vi "RampAcceleration.vi"(7 "Low Pass Filter Average Length\n(.003-.007 Rec)":dbl=0.05, 10 "Joystick Input":dbl(slide) scale=-1.0..1.0) -> (3 "Motor Output":dbl)   [LabVIEW 2013]
uses:
  <vilib>/ptbypt/NI_PtbyPt.lvlib
  <vilib>/addons/control/pid/NI_PID_pid.lvlib
  <vilib>/addons/control/pid/pid.llb/PID Output Rate Limiter (DBL).vi
panel:
  in  "output rate (EGU/min)":dbl=200.0
  in  "Average Filter Sample Length":i32=10
  out "Input to Motor":T1(graph)={"Joystick Input"=0.0, "upper limit"=-1.761109083191672e-27, "upper limit"=0.0, "output"=0.0}
  # "Credit to Team 3005"
  # "Lower means less responsive curve\nHigher means quick, more responsive"
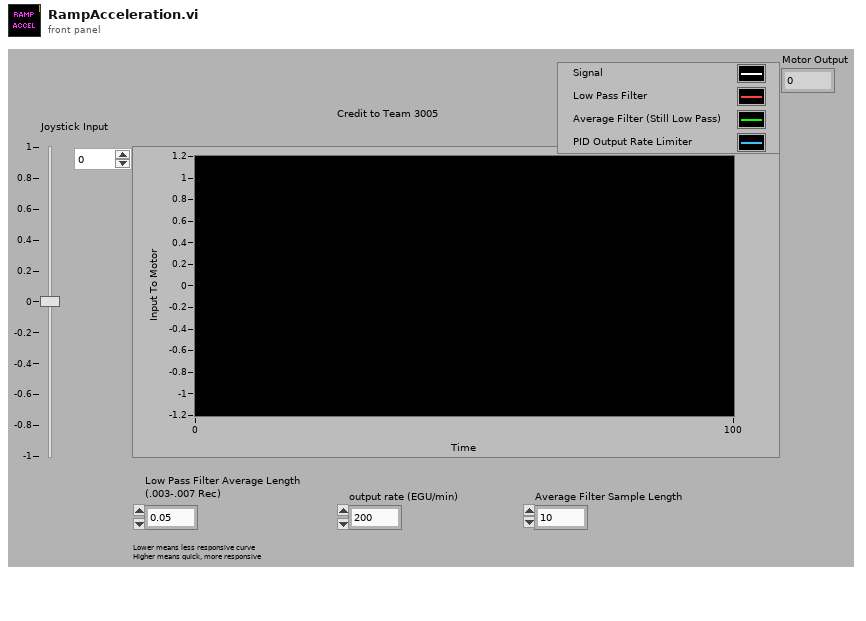
[diagram p1: front panel]
types:
  T1 = cluster{"Joystick Input":dbl, "upper limit":dbl, "upper limit":dbl, "output":dbl}
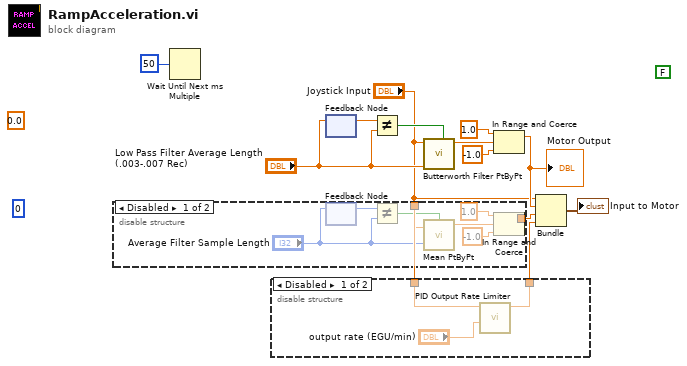
[diagram p0: block diagram]
diagram:
  (unwired) FALSE
  (unwired) 0 ("Average Filter Sample Length")
  (unwired) 0.0 ("Low Pass Filter Average Length")
  n1 = disable-structure shown="Disabled" {
    disable-tunnel: [w17 _] -> w6
    disable-tunnel: "Joystick Input" -> [w13 _]
    frame Disabled {
      n2 = feedback #1() -> (w16:i32)  [unwired: 1 in]
      n3 = feedback-in #1("Average Filter Sample Length") -> ()
      n4 = Not Equal?(x=w16, y="Average Filter Sample Length") -> (x != y?=w14:bool)
      n5 = call <vilib>:"Mean PtByPt.vi"("x"=w13, "sample length"="Average Filter Sample Length", "initialize"=w14) -> ("mean"=w18:dbl)  [unwired: 1 in, 1 out]
      n6 = In Range and Coerce(upper limit=1.0, x=w18, lower limit=-1.0) -> (coerced(x)=w17:dbl)  [unwired: 1 out]
    }
    frame Enabled {
    }
  }
  n7 = Wait Until Next ms Multiple(millisecond multiple=u32 50) -> ()  [unwired: 1 out]
  n8 = disable-structure shown="Disabled" {
    disable-tunnel: "Joystick Input" -> [w23 _]
    disable-tunnel: [w21 _] -> w1
    frame Disabled {
      n9 = call-poly <vilib>:"PID Output Rate Limiter.vi"("output rate (EGU/min)"="output rate (EGU/min)", "input (controller output)"=w23) -> ("output"=w21:dbl)  [unwired: 6 in, 1 out]
    }
    frame Enabled {
    }
  }
  n10 = feedback #2() -> (w5:dbl)  [unwired: 1 in]
  n11 = feedback-in #2("Low Pass Filter Average Length\n(.003-.007 Rec)") -> ()
  n12 = Not Equal?(x=w5, y="Low Pass Filter Average Length\n(.003-.007 Rec)") -> (x != y?=w3:bool)
  n13 = call <vilib>:"Butterworth Filter PtByPt.vi"("initialize"=w3, "low cutoff freq: fl"="Low Pass Filter Average Length\n(.003-.007 Rec)", "x"="Joystick Input") -> ("Filtered x"=w10:dbl)  [unwired: 6 in, 1 out]
  n14 = In Range and Coerce(upper limit=1.0, x=w10, lower limit=-1.0) -> (coerced(x)=w9:dbl)  [unwired: 1 out]
  "Motor Output" <- w9
  n15 = Bundle("Joystick Input"="Joystick Input", "upper limit"=w9, "upper limit"=w6, "output"=w1) -> (→"Input to Motor":T1)  [unwired: 1 in]
